vi "例5.6“初始化数组”函数.vi"() -> ()   [LabVIEW 2017]
panel:
  out "初始化的数组 2":dbl[][](array[numeric])
  out "初始化的数组":dbl[](array[numeric])
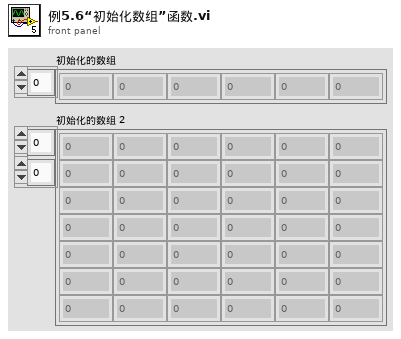
[diagram p1: front panel]
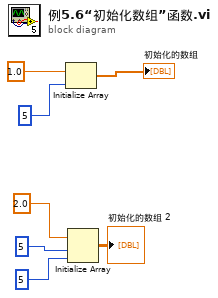
[diagram p0: block diagram]
diagram:
  n1 = Initialize Array(1.0 ("元素"), 5 ("维数大小")) -> (→"初始化的数组":dbl[])
  n2 = Initialize Array(2.0 ("元素"), 5 ("维数大小"), 5 ("维数大小")) -> (→"初始化的数组 2":dbl[][])
